vi "5 x Lesen Double.vi"(5 "Datenfluss (in)":bool, 8 "Fehler (Eingang, kein Fehler)":errorcluster, 9 "Factorysettings":path, 11 "appended path":path) -> (0 "Fehler (Ausgang)":errorcluster, 3 "Double (Ausgang)":dbl, 4 "Datenfluss (out)":bool)   [LabVIEW 2020, in "Konfig-Dateien.lvlib"]
uses:
  Konfig-Dateien.lvlib
  SysLog/SysLog Interface cRIO.ctl
  SysLog/SysLog_cRIO.lvlib
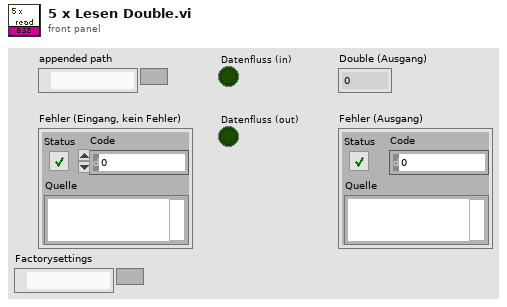
[diagram p1: front panel]
types:
  T1 = typedef "SysLog_cRIO.lvlib/SysLog Interface cRIO.ctl" = cluster{"FehlermeldungsCode":i32, "ErfolgsmeldungsCode":i32, "ParameterListenString":string, "intern":bool}
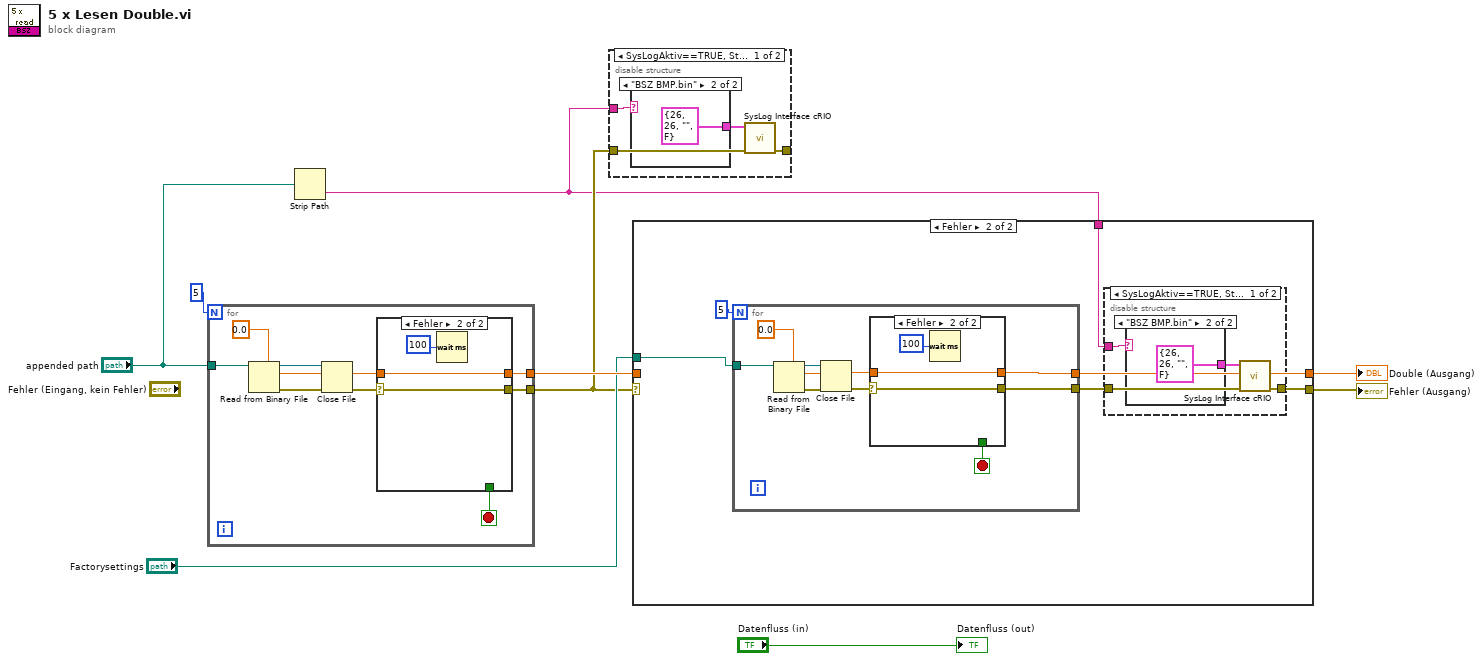
[diagram p0: block diagram]
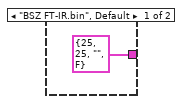
[diagram p2: hidden frame]
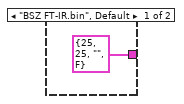
[diagram p5: hidden frame]
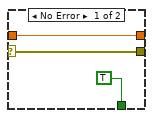
[diagram p7: hidden frame]
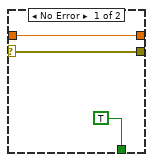
[diagram p8: hidden frame]
diagram:
  n1 = for {
    N: 5 -> [_]
    tunnel: "appended path" -> [w18]
    tunnel: [w14] -> w7
    tunnel: [w10] -> w2
    stop <- w17 stop-if-true
    n2 = Read from Binary File(5:0.0 ("Betriebsstunden FT-IR"), 11:w18) -> (0:w12:errorcluster, 2:w16:dbl, 3:w13:refnum<file>)  [unwired: 4 in, 1 out]
    n3 = Close File(refnum=w13, error in=w12) -> (error out=w11:errorcluster)  [unwired: 1 out]
    n4 = case shown="Fehler" w11 {
      selector: w11 -> [w19 w23]
      tunnel: [w19 w23] -> w10
      tunnel: [TRUE _] -> w17
      tunnel: [w20 w24] -> w14
      tunnel: w16 -> [w20 w24]
      frame No Error {
      }
      frame Error {
        n5 = Wait (ms)(milliseconds to wait=u32 100 ("Zu wartende ms")) -> ()  [unwired: 1 out]
      }
    }
  }
  n6 = Strip Path(path="appended path") -> (name=w1:string)  [unwired: 1 out]
  n7 = disable-structure shown="SysLogAktiv==TRUE, Standard" {
    disable-tunnel: w1 -> [w28 _]
    disable-tunnel: [w26 w31] -> _
    disable-tunnel: w2 -> [w25 w31]
    frame condition #0 (active) {
      n8 = case shown="\"BSZ BMP.bin\"" w28 {
        tunnel: [T1 {"FehlermeldungsCode"=25, "ErfolgsmeldungsCode"=25, "ParameterListenString"="", "intern"=FALSE} ("Cluster (in)") T1 {"FehlermeldungsCode"=26, "ErfolgsmeldungsCode"=26, "ParameterListenString"="", "intern"=FALSE} ("Cluster (in)")] -> w27
        frame "BSZ FT-IR.bin", Default {
        }
        frame "BSZ BMP.bin" {
        }
      }
      n9 = call "SysLog Interface cRIO.vi"("Fehler (in)"=w25, "Cluster (in)"=w27) -> ("Fehler (Ausgang)"=w26:errorcluster)  [unwired: 9 in]
    }
    frame condition #1 {
    }
  }
  n10 = case shown="Fehler" w2 {
    selector: w2 -> [w33 _]
    tunnel: [w33 w36] -> w4
    tunnel: w7 -> [w32 _]
    tunnel: [w32 w35] -> w6
    tunnel: "Factorysettings" -> [_ w38]
    tunnel: w1 -> [_ w34]
    frame No Error {
    }
    frame Error {
      n11 = for {
        N: 5 -> [_]
        tunnel: w38 -> [w55]
        tunnel: [w51] -> w35
        tunnel: [w47] -> w37
        stop <- w54 stop-if-true
        n12 = Read from Binary File(5:0.0 ("Betriebsstunden FT-IR"), 11:w55) -> (0:w49:errorcluster, 2:w53:dbl, 3:w50:refnum<file>)  [unwired: 4 in, 1 out]
        n13 = Close File(refnum=w50, error in=w49) -> (error out=w48:errorcluster)  [unwired: 1 out]
        n14 = case shown="Fehler" w48 {
          selector: w48 -> [w56 w60]
          tunnel: [w56 w60] -> w47
          tunnel: [TRUE _] -> w54
          tunnel: [w57 w61] -> w51
          tunnel: w53 -> [w57 w61]
          frame No Error {
          }
          frame Error {
            n15 = Wait (ms)(milliseconds to wait=u32 100 ("Zu wartende ms")) -> ()  [unwired: 1 out]
          }
        }
      }
      n16 = disable-structure shown="SysLogAktiv==TRUE, Standard" {
        disable-tunnel: w34 -> [w43 _]
        disable-tunnel: [w41 w46] -> w36
        disable-tunnel: w37 -> [w40 w46]
        frame condition #0 (active) {
          n17 = case shown="\"BSZ BMP.bin\"" w43 {
            tunnel: [T1 {"FehlermeldungsCode"=25, "ErfolgsmeldungsCode"=25, "ParameterListenString"="", "intern"=FALSE} ("Cluster (in)") T1 {"FehlermeldungsCode"=26, "ErfolgsmeldungsCode"=26, "ParameterListenString"="", "intern"=FALSE} ("Cluster (in)")] -> w42
            frame "BSZ FT-IR.bin", Default {
            }
            frame "BSZ BMP.bin" {
            }
          }
          n18 = call "SysLog Interface cRIO.vi"("Fehler (in)"=w40, "Cluster (in)"=w42) -> ("Fehler (Ausgang)"=w41:errorcluster)  [unwired: 9 in]
        }
        frame condition #1 {
        }
      }
    }
  }
  "Fehler (Ausgang)" <- w4
  "Double (Ausgang)" <- w6
  "Datenfluss (out)" <- "Datenfluss (in)"
